vi "Visa_Write read_UI GETPORT.vi"(0 "Cypress in":refnum<class "Cypress.lvclass">, 1 "VISA resource name":refnum<visa-resource-name>, 2 "Command to Send":string, 3 "Expected Response":string, 4 "Buttons":bool[](array[boolean]), 5 "error in (no error)":errorcluster) -> (14 "Cypress out":refnum<class "Cypress.lvclass">, 15 "VISA Refnum out":refnum<visa-resource-name>, 16 "Expected Response out":string, 17 "Port":string, 19 "error out":errorcluster)   [LabVIEW 2020, in "Cypress.lvclass"]
uses:
  Cypress.lvclass
  Abstract/Serial Device/Combo Box Devices.ctl
  Abstract/Serial Device/Combo Box Comandos.ctl
  UI Actor/UI Actor.lvclass
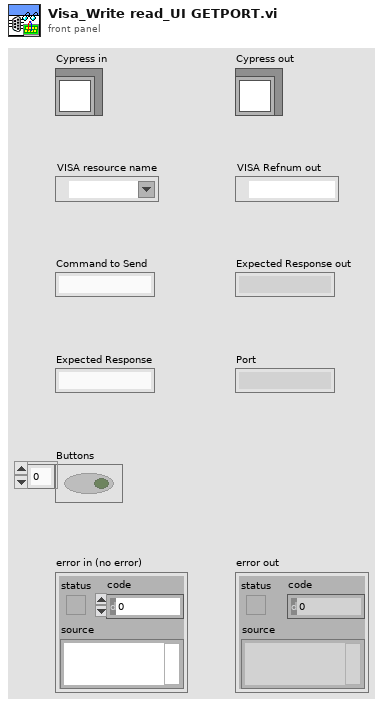
[diagram p1: front panel]
types:
  T1 = typedef "Combo Box Comandos.ctl" = string
  T2 = typedef "Combo Box Devices.ctl" = string
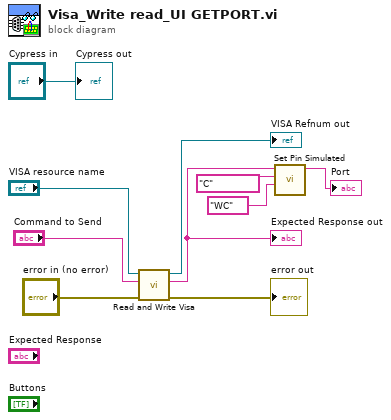
[diagram p0: block diagram]
diagram:
  n1 = call "Read and Write Visa.vi"("error in (no error)"="error in (no error)", "Command to Send"="Command to Send", "VISA Refnum in"="VISA resource name") -> ("error out"=→"error out":errorcluster, "Expected Response out"=w1:string, "VISA Refnum out"=→"VISA Refnum out":refnum<visa-resource-name>)  [unwired: 6 in]
  "Expected Response out" <- w1
  n2 = call "Set Pin Simulated.vi"("Command"=T1 "WC", "Serial Devide Brand"=T2 "C", "Command to Send"=w1) -> ("Puerto"=→"Port":string)  [unwired: 6 in, 2 out]
  "Cypress out" <- "Cypress in"
